vi "Limited number writer.vi"() -> ()   [LabVIEW 2025]
uses:
  <vilib>/xnet/xnet.llb/XNET Frame Type Ethernet.ctl
  <vilib>/xnet/xnet.llb/XNET Create Session (Frame Output Stream).vi
  <vilib>/xnet/xnet.llb/XNET Write (Frame Ethernet).vi
  <vilib>/xnet/xnet.llb/XNET Create Session (Frame Input Stream).vi
  <vilib>/xnet/xnet.llb/XNET Write (State Ethernet Sleep).vi
  <vilib>/xnet/xnet.llb/XNET Write (State Ethernet Wake).vi
  Automotive Ethernet Bus Monitor/Automotive Ethernet Bus Monitor.lvclass
  <resource>/objmgr/xnet.rc
panel:
  out "Number of Frames Sent":i32
  in  "Stop VI":bool
  in  "Start":bool
  in  "Stop":bool
  in  "Interface":refnum<k21>="ENET1"
  in  "Test Type":T1(tab)
  out "Multi Message Test Error":errorcluster
  in  "Ethertype 1":u16=1 format="%.0x"
  in  "payload 2":string="payload1"
  in  "Ethertype 3":u16=3 format="%.0x"
  in  "payload 3":string="medium payload"
  in  "Ethertype 2":u16=2 format="%.0x"
  in  "payload 1":string="payload2 is so much longer than payload1"
  in  "priority  2":u8=3
  in  "VID 3":u16=2
  in  "Has VLAN Tag 3":bool=TRUE
  in  "destination MAC address  2":cluster{u8, u8, u8, u8, u8, u8}={255, 255, 255, 255, 255, 255} {"?" format="%.0x"; "?" format="%.0x"; "?" format="%.0x"; "?" format="%.0x"; "?" format="%.0x"; "?" format="%.0x"}
  in  "Number of messages":i32
  in  "Ethertype":u16=1 format="%.0x"
  in  "priority":u8=3
  in  "VID 2":u16=2
  in  "Has VLAN Tag 2":bool=TRUE
  in  "destination MAC address":cluster{u8, u8, u8, u8, u8, u8}={255, 255, 255, 255, 255, 255} {"?" format="%.0x"; "?" format="%.0x"; "?" format="%.0x"; "?" format="%.0x"; "?" format="%.0x"; "?" format="%.0x"}
  out "Single Packet Stream Error":errorcluster
  in  "milliseconds between messages":u32=2
  out "Sleep Capability":u32(ring) items=["Disabled / Not Available", "Enabled"]
  out "PHY Power Mode":u32(ring) items=["Normal", "Sleep"]
  out "Wake Up Request Count":u64
  out "Wake Up Pulse Count":u64
  out "Low Power Sleep Count":u64
  out "Operational Status":u32(ring) items=["Down", "Up"]
  in  "Sleep":bool
  in  "Wake":bool
  out "TC10 Error":errorcluster
  # "VI used for testing packets in the Auto Ethernet Bus Monitor"
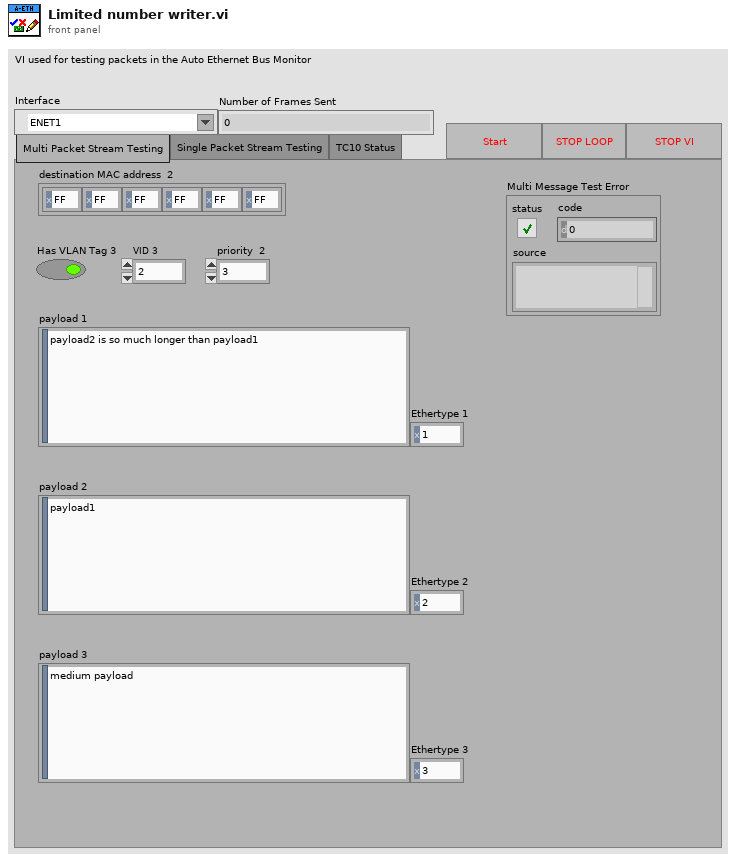
[diagram p1: front panel]
types:
  T1 = enum32{"Multi Packet Stream Testing", "Single Packet Stream Testing", "TC10 Status"}
  T2 = typedef "XNET Frame Type Ethernet.ctl" = u16
  T3 = cluster{"local timestamp":timestamp, "network timestamp":timestamp, "frame data":u8[], "fcs":u32, "type":T2, "network synced?":bool, "receive?":bool, "transmit?":bool, "error?":bool}
  T4 = cluster{"destination MAC address":cluster{u8, u8, u8, u8, u8, u8}, "source MAC address":cluster{u8, u8, u8, u8, u8, u8}, "Has VLAN Tag":bool, "VLAN Tag":cluster{"TPID":u16, "priority":u8, "DEI":bool, "VID":u16}, "Ethertype":u16}
  T5 = cluster{"TPID":u16, "priority":u8, "DEI":bool, "VID":u16}
  T6 = cluster{"local timestamp":timestamp, "network timestamp":timestamp, "frame data":u8[], "fcs":u32, "type":T2, "network synced?":bool, "receive?":bool, "transmit?":bool, "error?":bool}[]
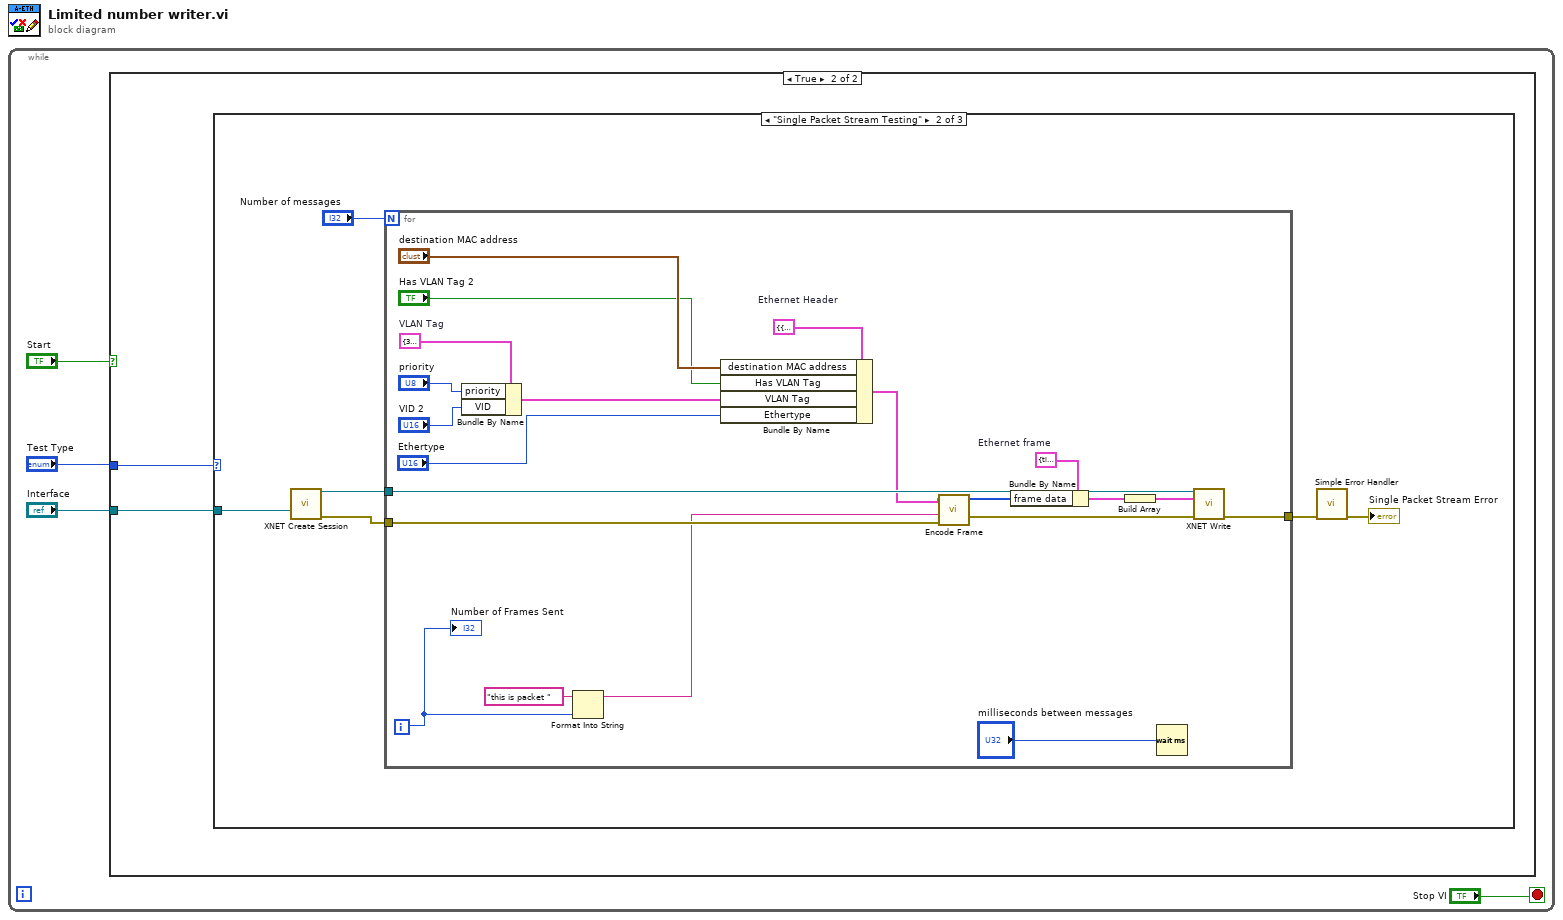
[diagram p0: block diagram]
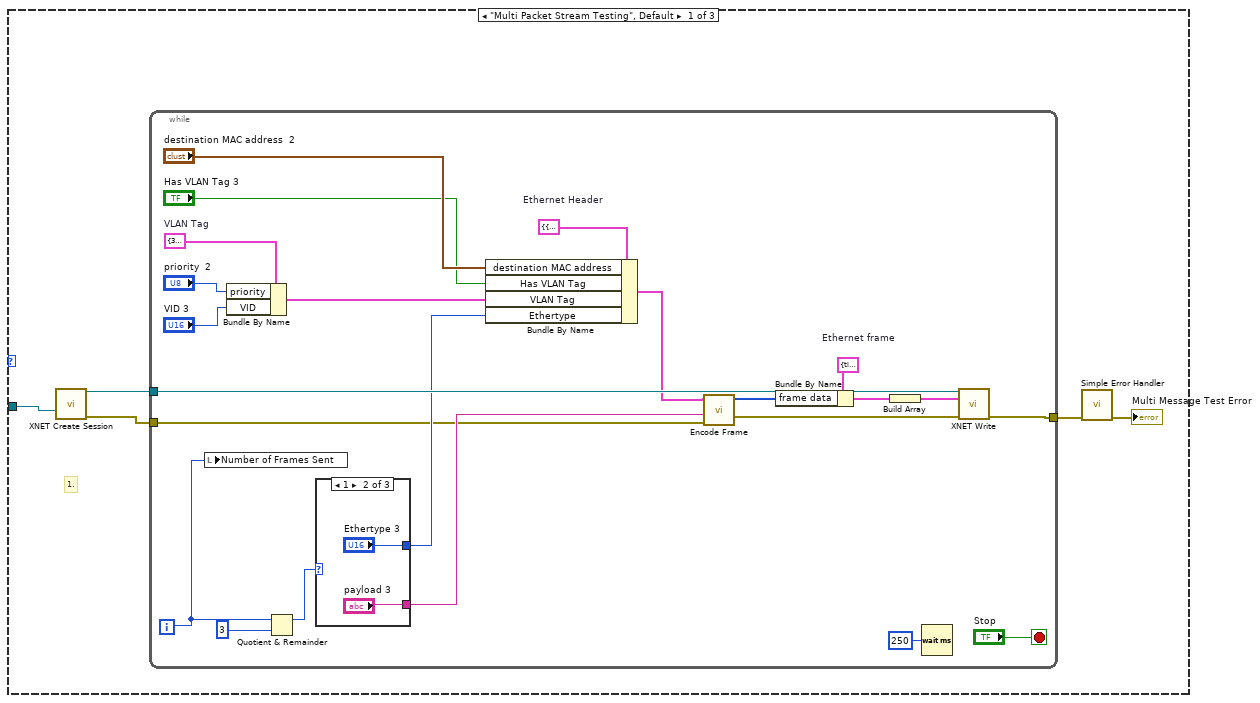
[diagram p3: hidden frame]
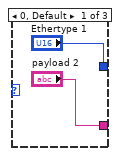
[diagram p4: hidden frame]
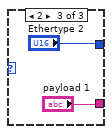
[diagram p5: hidden frame]
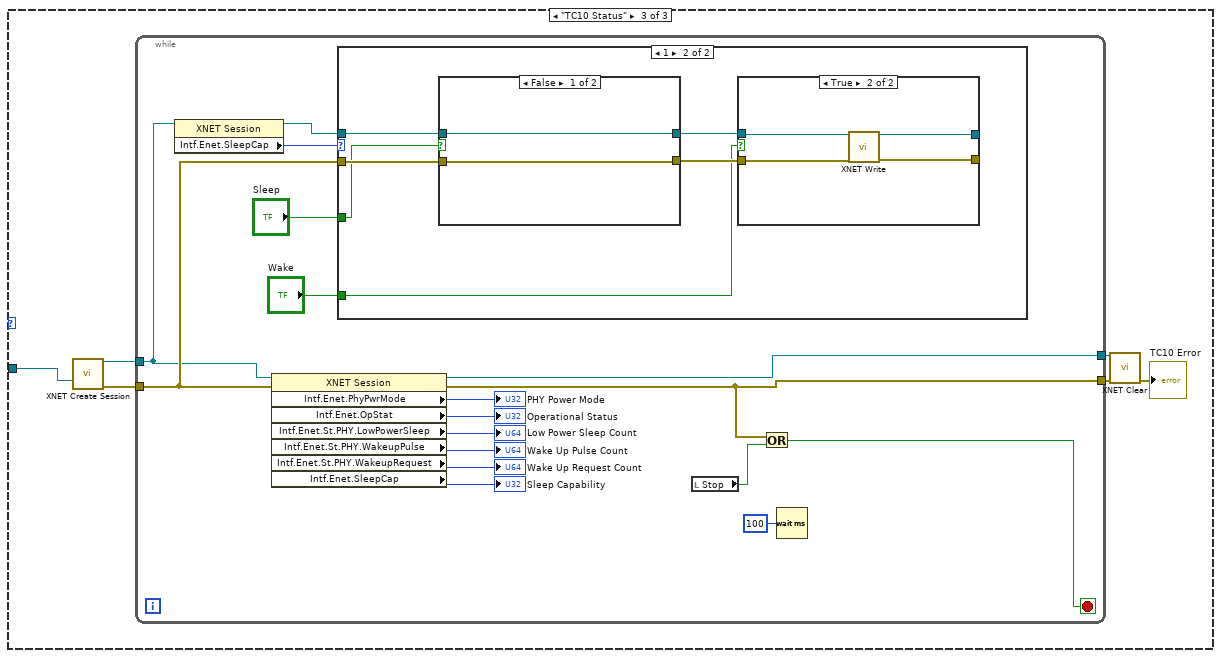
[diagram p6: hidden frame]
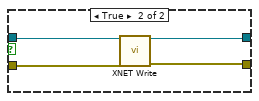
[diagram p8: hidden frame]
diagram:
  n1 = while {
    stop <- "Stop VI" stop-if-true
    n2 = case shown="True" "Start" {
      tunnel: "Interface" -> [_ w6]
      tunnel: "Test Type" -> [_ w5]
      frame False {
      }
      frame True {
        n3 = case shown="\"Single Packet Stream Testing\"" w5 {
          tunnel: w6 -> [w7 w46 w73]
          frame "Multi Packet Stream Testing", Default {
            # "1."
            n4 = call-poly <vilib>:"XNET Create Session.vi"("interface"=w7) -> ("session out"=w8:refnum<k21>, "error out"=w10:errorcluster)  [unwired: 13 in]
            n5 = while {
              tunnel: w8 -> [w34]
              tunnel: [w31] -> w9
              tunnel: w10 -> [w13]
              i -> [w12]
              stop <- "Stop" stop-if-true
              w25 = T3 {"local timestamp"=timestamp(0 s since 1904-01-01), "network timestamp"=timestamp(0 s since 1904-01-01), "frame data"=[], "fcs"=0, "type"=0, "network synced?"=FALSE, "receive?"=FALSE, "transmit?"=FALSE, "error?"=FALSE}  # Ethernet frame
              w30 = T4 {"destination MAC address"={0, 0, 0, 0, 0, 0}, "source MAC address"={0, 0, 0, 0, 0, 0}, "Has VLAN Tag"=FALSE, "VLAN Tag"={"TPID"=33024, "priority"=0, "DEI"=FALSE, "VID"=0}, "Ethertype"=0}  # Ethernet Header
              w29 = T5 {"TPID"=33024, "priority"=0, "DEI"=FALSE, "VID"=0}  # VLAN Tag
              n6 = local write "Number of Frames Sent"(w12) -> ()
              n7 = Bundle By Name(cluster=w29, "priority"="priority  2", "VID"="VID 3") -> (w28:T5)
              n8 = Quotient & Remainder(x=w12, y=3) -> (x-y*floor(x/y)=w20:i32)  [unwired: 1 out]
              n9 = case shown="1" w20 {
                tunnel: ["payload 2" "payload 3" "payload 1"] -> w15
                tunnel: ["Ethertype 1" "Ethertype 3" "Ethertype 2"] -> w18
                frame 0, Default {
                }
                frame 1 {
                }
                frame 2 {
                }
              }
              n10 = Bundle By Name(cluster=w30, "destination MAC address"="destination MAC address  2", "Has VLAN Tag"="Has VLAN Tag 3", "VLAN Tag"=w28, "Ethertype"=w18) -> (w17:T4)
              n11 = call "Encode Frame.vi"("error in (no error)"=w13, "payload"=w15, "Ethernet Header"=w17) -> ("error out"=w14:errorcluster, "frame data"=w16:u8[])  [unwired: 7 in]
              n12 = Bundle By Name(cluster=w25, "frame data"=w16) -> (w24:T3)
              n13 = Build Array(w24) -> (w23:T6)
              n14 = Wait (ms)(milliseconds to wait=u32 250) -> ()  [unwired: 1 out]
              n15 = call-poly <vilib>:"XNET Write.vi"("session in"=w34, "data"=w23, "error in (no error)"=w14) -> ("error out"=w31:errorcluster)  [unwired: 11 in, 1 out]
            }
            n16 = call <vilib>:"Simple Error Handler.vi"("error in (no error)"=w9) -> ("error out"=→"Multi Message Test Error":errorcluster)  [unwired: 4 in, 4 out]
          }
          frame "Single Packet Stream Testing" {
            n17 = call-poly <vilib>:"XNET Create Session.vi"("interface"=w46) -> ("session out"=w45:refnum<k21>, "error out"=w43:errorcluster)  [unwired: 13 in]
            n18 = for {
              N: "Number of messages" -> [_]
              tunnel: w45 -> [w67]
              tunnel: [w64] -> w44
              tunnel: w43 -> [w51]
              i -> [w49]
              w58 = T3 {"local timestamp"=timestamp(0 s since 1904-01-01), "network timestamp"=timestamp(0 s since 1904-01-01), "frame data"=[], "fcs"=0, "type"=0, "network synced?"=FALSE, "receive?"=FALSE, "transmit?"=FALSE, "error?"=FALSE}  # Ethernet frame
              w63 = T4 {"destination MAC address"={0, 0, 0, 0, 0, 0}, "source MAC address"={0, 0, 0, 0, 0, 0}, "Has VLAN Tag"=FALSE, "VLAN Tag"={"TPID"=33024, "priority"=0, "DEI"=FALSE, "VID"=0}, "Ethertype"=0}  # Ethernet Header
              w62 = T5 {"TPID"=33024, "priority"=0, "DEI"=FALSE, "VID"=0}  # VLAN Tag
              n19 = Bundle By Name(cluster=w62, "priority"="priority", "VID"="VID 2") -> (w61:T5)
              n20 = Format Into String(initial string="this is packet ", w49) -> (resulting string=w48:string)  [unwired: 2 in, 1 out]
              n21 = Bundle By Name(cluster=w63, "destination MAC address"="destination MAC address", "Has VLAN Tag"="Has VLAN Tag 2", "VLAN Tag"=w61, "Ethertype"="Ethertype") -> (w54:T4)
              n22 = call "Encode Frame.vi"("error in (no error)"=w51, "payload"=w48, "Ethernet Header"=w54) -> ("error out"=w52:errorcluster, "frame data"=w53:u8[])  [unwired: 7 in]
              n23 = Bundle By Name(cluster=w58, "frame data"=w53) -> (w57:T3)
              n24 = Build Array(w57) -> (w56:T6)
              n25 = Wait (ms)(milliseconds to wait="milliseconds between messages") -> ()  [unwired: 1 out]
              n26 = call-poly <vilib>:"XNET Write.vi"("session in"=w67, "data"=w56, "error in (no error)"=w52) -> ("error out"=w64:errorcluster)  [unwired: 11 in, 1 out]
              "Number of Frames Sent" <- w49
            }
            n27 = call <vilib>:"Simple Error Handler.vi"("error in (no error)"=w44) -> ("error out"=→"Single Packet Stream Error":errorcluster)  [unwired: 4 in, 4 out]
          }
          frame "TC10 Status" {
            n28 = call-poly <vilib>:"XNET Create Session.vi"("interface"=w73) -> ("session out"=w71:refnum<k21>, "error out"=w72:errorcluster)  [unwired: 13 in]
            n29 = while {
              tunnel: w72 -> [w90]
              tunnel: w71 -> [w86]
              tunnel: [w75] -> w69
              tunnel: [w74] -> w68
              stop <- w76 stop-if-true
              n30 = property class="XNET Session"(reference=w86) -> (reference out=w85:refnum<k21>, "Intf.Enet.SleepCap"=w87:u32)  [unwired: 1 in, 1 out]
              n31 = property class="XNET Session"(reference=w86, error in=w90) -> (reference out=w75:refnum<k21>, error out=w74:errorcluster, "Intf.Enet.PhyPwrMode"=→"PHY Power Mode":u32, "Intf.Enet.OpStat"=→"Operational Status":u32, "Intf.Enet.St.PHY.LowPowerSleep"=→"Low Power Sleep Count":u64, "Intf.Enet.St.PHY.WakeupPulse"=→"Wake Up Pulse Count":u64, "Intf.Enet.St.PHY.WakeupRequest"=→"Wake Up Request Count":u64, "Intf.Enet.SleepCap"=→"Sleep Capability":u32)
              n32 = case shown="1" w87 {
                tunnel: w85 -> [_ w96]
                tunnel: w90 -> [_ w93]
                tunnel: "Sleep" -> [_ w92]
                tunnel: "Wake" -> [_ w91]
                frame 0, Default {
                }
                frame 1 {
                  n33 = case shown="False" w92 {
                    tunnel: w96 -> [w98 w102]
                    tunnel: w93 -> [w97 w101]
                    tunnel: [w98 w100] -> w95
                    tunnel: [w97 w99] -> w94
                    frame False {
                    }
                    frame True {
                      n34 = call-poly <vilib>:"XNET Write.vi"("session in"=w102, "error in (no error)"=w101) -> ("session out"=w100:refnum<k21>, "error out"=w99:errorcluster)  [unwired: 12 in]
                    }
                  }
                  n35 = case shown="True" w91 {
                    tunnel: w95 -> [w104 w108]
                    tunnel: w94 -> [w103 w107]
                    tunnel: [w104 w106] -> _
                    tunnel: [w103 w105] -> _
                    frame False {
                    }
                    frame True {
                      n36 = call-poly <vilib>:"XNET Write.vi"("session in"=w108, "error in (no error)"=w107) -> ("session out"=w106:refnum<k21>, "error out"=w105:errorcluster)  [unwired: 12 in]
                    }
                  }
                }
              }
              n37 = local read "Stop"() -> (w77:bool)
              n38 = Or(x=w74, y=w77) -> (x .or. y?=w76:bool)
              n39 = Wait (ms)(milliseconds to wait=u32 100) -> ()  [unwired: 1 out]
            }
            n40 = call <vilib>:"XNET Clear.vi"("session in"=w69, "error in (no error)"=w68) -> ("error out"=→"TC10 Error":errorcluster)  [unwired: 13 in]
          }
        }
      }
    }
  }
